vi "Global.vi"() -> ()   [LabVIEW 2020]
panel:
  out "合格状态":bool
  out "判定长度":i32
  in  "最大值判定参数":T1
  in  "产品型号引用":refnum<vi>
  in  "产品追溯码引用":refnum<vi>
  out "产品追溯码":string
  in  "Str引用句柄":refnum<vi>
  in  "上序状态颜色":refnum<vi>
  out "硬件版本号":string
  out "软件版本号":string
  out "逆向空载系数":dbl
  in  "STOP_NVH":bool
  in  "联机模式":enum16{"单机", "追溯"}(ring)=enum."追溯"
  out "用户信息":T2
  out "产品型号":string
  out "传感器读数":T3 {"吸收电流" format="%#.3f"; "输出扭矩(大)" format="%#.3f"; "输出扭矩(小)" format="%#.3f"; "输入扭矩" format="%#.3f"; "输入编码位移" format="%#.3f"; "工装移载位移" format="%#.3f"; "输入移载位移" format="%#.3f"; "输入旋转位移" format="%#.3f"}
  out "设备状态":i16
  in  "CAN Info":T4={"波特率"=11, "ID"=0, "帧类型"=enum."标准帧", "帧格式"=enum."数据帧", "周期(ms)"=10} {"周期(ms)" min=1 format="%d ms"; "ID" format="0x%x"; "波特率" items=["5Kbps", "10Kbps", "20Kbps", "40Kbps", "50Kbps", "80Kbps", "100Kbps", "125Kbps", "200Kbps", "250Kbps", "400Kbps", "500Kbps", "666Kbps", "800Kbps", "1000Kbps"]}
  in  "输出占空比":refnum<vi>
  out "spectrum info":void[](array[numeric])
  in  "波特率":T5(ring)=enum."500Kbps"
  in  "CAN_CYCLE":T6(array[cluster]) {"周期(ms)" min=1 format="%d ms"; "ID" format="0x%x"}
  in  "启用CAN":bool
  in  "STOP_CAN":bool
  in  "复检判定参数":T7
  out "工位二扭矩偏移":cluster{"正向":dbl, "逆向":dbl}
  out "工位一扭矩偏移":cluster{"正向":dbl, "逆向":dbl}
  out "复检参数":cluster{"复检速度":dbl, "换向扭矩":dbl}
  out "扭矩":cluster{"工位一":dbl, "工位二":dbl}
  out "T2":dbl
  out "T1":dbl
  in  "占空比采集":bool
  out "S7 Link":refnum<k5>
  out "产品编号":string
  in  "计时开始":bool
  in  "计时复位":bool
  in  "IO_Stop":bool
  in  "合格数量":i32
  in  "生产数量":i32
  in  "试验项目":bool[](array[boolean])
  out "模式":u32
  in  "更换产品":refnum<vi>
  in  "提示信息":refnum<vi>
  in  "程序自动":refnum<vi>
  in  "报警图标":refnum<vi>
  in  "程序关闭":bool
  in  "Info":refnum<vi>
  in  "Result":refnum<vi>
  in  "批次":refnum<vi>
  # "帧ID"
  # "帧类型"
  # "帧格式"
  # "帧数据"
  # "周期"
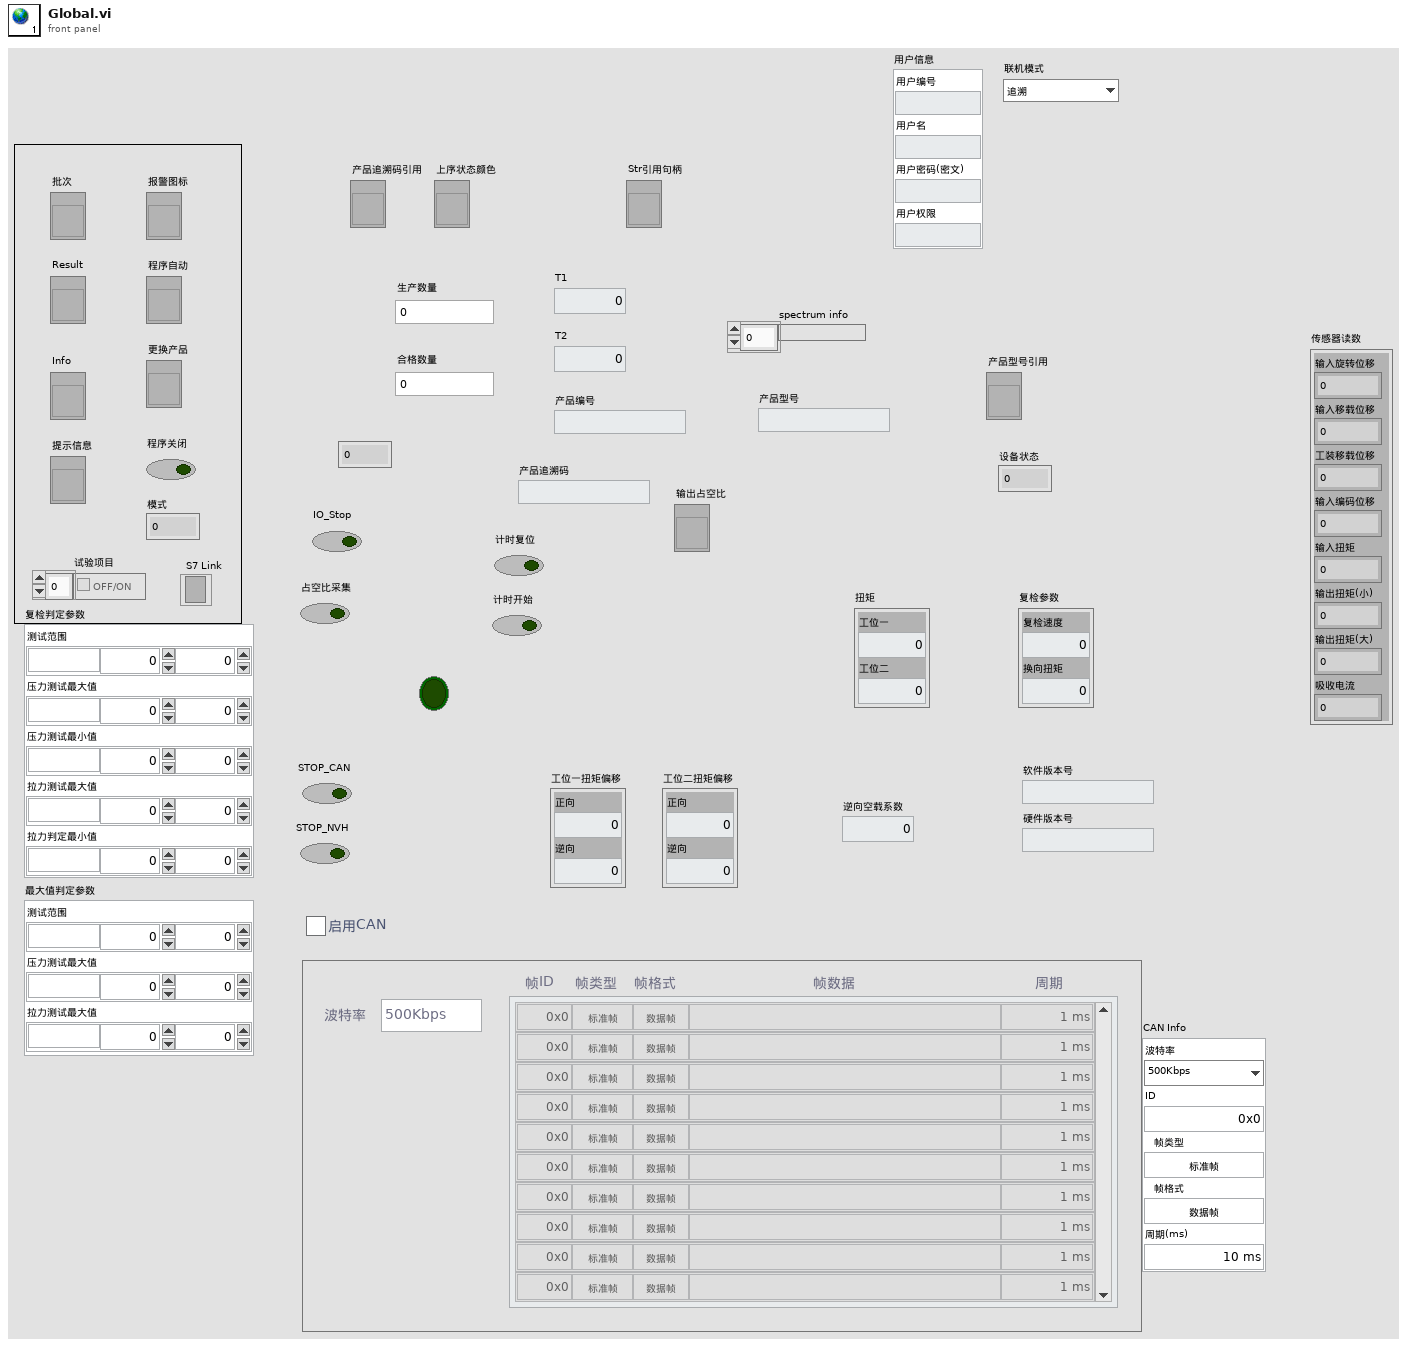
[diagram p1: front panel]
types:
  T1 = cluster{"测试范围":cluster{"单位":string, "下限":dbl, "上限":dbl}, "压力测试最大值":cluster{"单位":string, "下限":dbl, "上限":dbl}, "拉力测试最大值":cluster{"单位":string, "下限":dbl, "上限":dbl}}
  T2 = cluster{"用户编号":string, "用户名":string, "用户密码(密文)":string, "用户权限":string}
  T3 = cluster{"输入旋转位移":sgl, "输入移载位移":sgl, "工装移载位移":sgl, "输入编码位移":sgl, "输入扭矩":sgl, "输出扭矩(小)":sgl, "输出扭矩(大)":sgl, "吸收电流":sgl}
  T4 = cluster{"波特率":u32, "ID":u32, "帧类型":enum8{"标准帧", "扩展帧"}, "帧格式":enum16{"数据帧", "远程帧"}, "周期(ms)":u32}
  T5 = enum16{"5Kbps", "10Kbps", "20Kbps", "40Kbps", "50Kbps", "80Kbps", "100Kbps", "125Kbps", "200Kbps", "250Kbps", "400Kbps", "500Kbps", "666Kbps", "800Kbps", "1000Kbps"}
  T6 = cluster{"ID":u32, "帧类型":enum8{"标准帧", "扩展帧"}, "帧格式":enum16{"数据帧", "远程帧"}, "帧数据":string, "周期(ms)":u32}[]
  T7 = cluster{"测试范围":cluster{"单位":string, "下限":dbl, "上限":dbl}, "压力测试最大值":cluster{"单位":string, "下限":dbl, "上限":dbl}, "压力测试最小值":cluster{"单位":string, "下限":dbl, "上限":dbl}, "拉力测试最大值":cluster{"单位":string, "下限":dbl, "上限":dbl}, "拉力判定最小值":cluster{"单位":string, "下限":dbl, "上限":dbl}}
diagram:
